vi "password.vi"() -> ()   [LabVIEW 2023]
panel:
  in  "Boolean 2":bool
  out "Boolean":bool
  in  "String 2":string
  in  "String":string
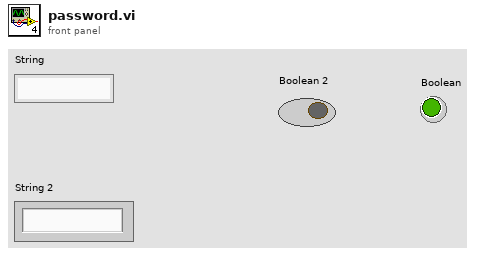
[diagram p1: front panel]
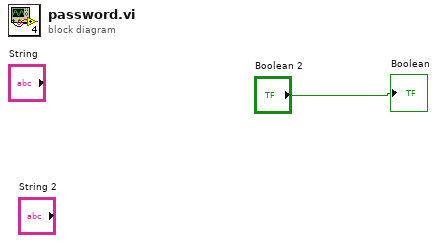
[diagram p0: block diagram]
diagram:
  "Boolean" <- "Boolean 2"
